vi "parse_map_data.vi"(4 "error in":errorcluster, 6 "Array?":bool, 7 "Map":string) -> (0 "error out":errorcluster, 2 "Map Geojson":string, 3 "Lanes":cluster{"x":dbl[], "y":dbl[], "z":dbl[]})   [LabVIEW 2019, in "Lib_Simx.lvlib"]
doc: "Parse the map information depending on if this is in array format or GeoJSON format."
uses:
  Lib_Simx.lvlib
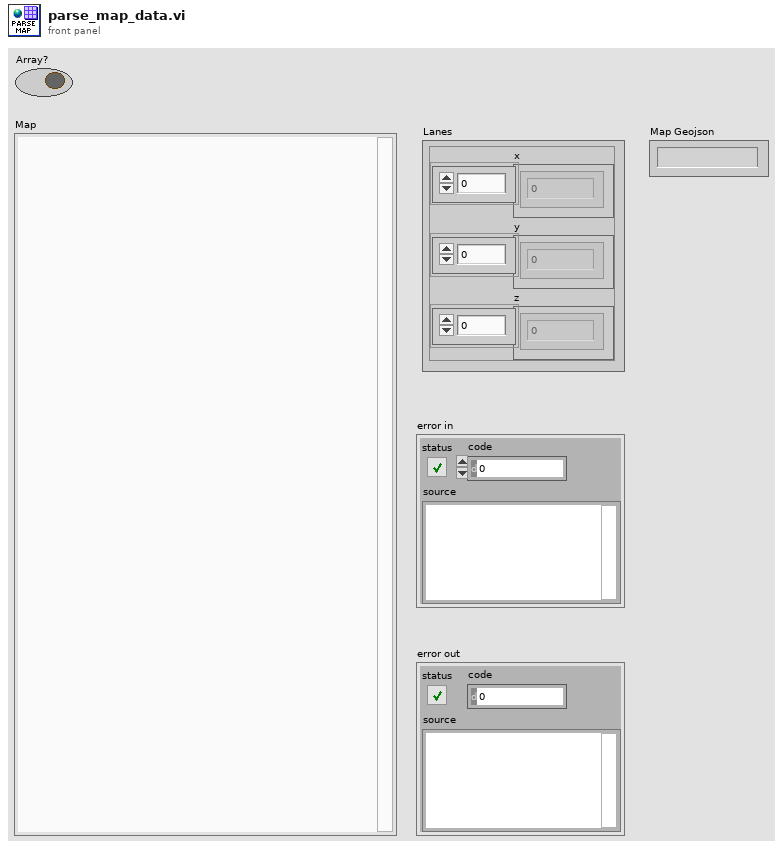
[diagram p1: front panel]
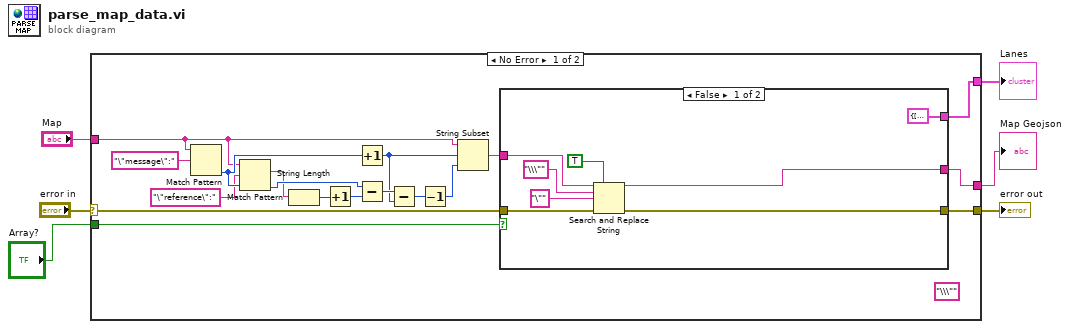
[diagram p0: block diagram]
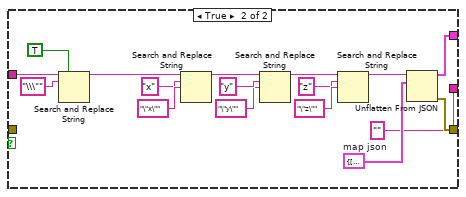
[diagram p2: hidden frame]
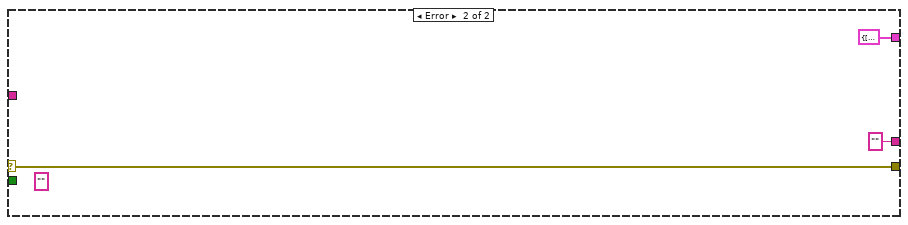
[diagram p3: hidden frame]
diagram:
  n1 = case shown="No Error" "error in" {
    selector: "error in" -> [w8 w52]
    tunnel: "Map" -> [w16 _]
    tunnel: [w15 w52] -> w5
    tunnel: [w10 cluster{"x":dbl[], "y":dbl[], "z":dbl[]} {"x"=[], "y"=[], "z"=[]} ("map json")] -> w3
    tunnel: [w9 "" ("result string")] -> w2
    tunnel: "Array?" -> [w7 _]
    frame No Error {
      (unwired) "\\\"" ("search string")
      n2 = Match Pattern(string=w16, regular expression="\"message\":") -> (offset past match=w24:i32)  [unwired: 1 in, 3 out]
      n3 = Match Pattern(string=w16, regular expression="\"reference\":", offset (0)=w24) -> (match substring=w19:string, offset past match=w22:i32)  [unwired: 2 out]
      n4 = String Length(string=w19) -> (length=w20:i32)
      n5 = Increment(x=w20) -> (x+1=w23:i32)
      n6 = Increment(x=w24) -> (x+1=w13:i32)
      n7 = Subtract(x=w22, y=w23) -> (x-y=w21:i32)
      n8 = Subtract(x=w21, y=w13) -> (x-y=w12:i32)
      n9 = Decrement(x=w12) -> (x-1=w11:i32)
      n10 = String Subset(string=w16, offset (0)=w13, length (rest)=w11) -> (substring=w14:string)
      n11 = case shown="False" w7 {
        tunnel: [w27 w49] -> w15
        tunnel: w14 -> [w29 w47]
        tunnel: [cluster{"x":dbl[], "y":dbl[], "z":dbl[]} {"x"=[], "y"=[], "z"=[]} ("map json") w34] -> w10
        tunnel: [w28 "" ("result string")] -> w9
        tunnel: w8 -> [w26 _]
        frame False {
          n12 = Search and Replace String(replace all?=TRUE ("replace all? (F)"), input string=w29, search string="\\\"", replace string="\"" ("replace string (\"\")"), error in=w26) -> (result string=w28:string, error out=w27:errorcluster)  [unwired: 3 in, 2 out]
        }
        frame True {
          w48 = cluster{"x":dbl[], "y":dbl[], "z":dbl[]} {"x"=[], "y"=[], "z"=[]}  # map json
          n13 = Search and Replace String(replace all?=TRUE ("replace all? (F)"), input string=w47, search string="\\\"") -> (result string=w42:string)  [unwired: 5 in, 3 out]
          n14 = Search and Replace String(input string=w42, search string="x", replace string="\"x\"" ("search string")) -> (result string=w41:string)  [unwired: 5 in, 3 out]
          n15 = Search and Replace String(input string=w41, search string="y", replace string="\"y\"" ("search string")) -> (result string=w36:string)  [unwired: 5 in, 3 out]
          n16 = Search and Replace String(input string=w36, search string="z", replace string="\"z\"" ("search string")) -> (result string=w35:string)  [unwired: 5 in, 3 out]
          n17 = Unflatten From JSON(JSON string=w35, type and defaults=w48) -> (value=w34:cluster{"x":dbl[], "y":dbl[], "z":dbl[]}, error out=w49:errorcluster)  [unwired: 5 in]
        }
      }
    }
    frame Error {
      (unwired) "" ("data out")
    }
  }
  "error out" <- w5
  "Lanes" <- w3
  "Map Geojson" <- w2
